vi "Setup User Messages.vi"(7 "Map Or Menu Ref":refnum<vi>, 8 "error in (no error)":errorcluster, 10 "Prev String Ref":refnum<vi>, 11 "String Ref":refnum<vi>) -> (0 "Error Out":errorcluster)   [LabVIEW 2014]
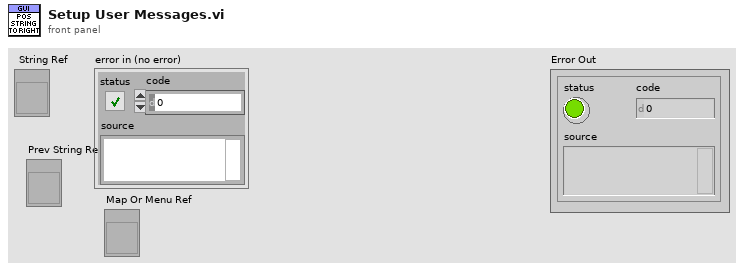
[diagram p1: front panel]
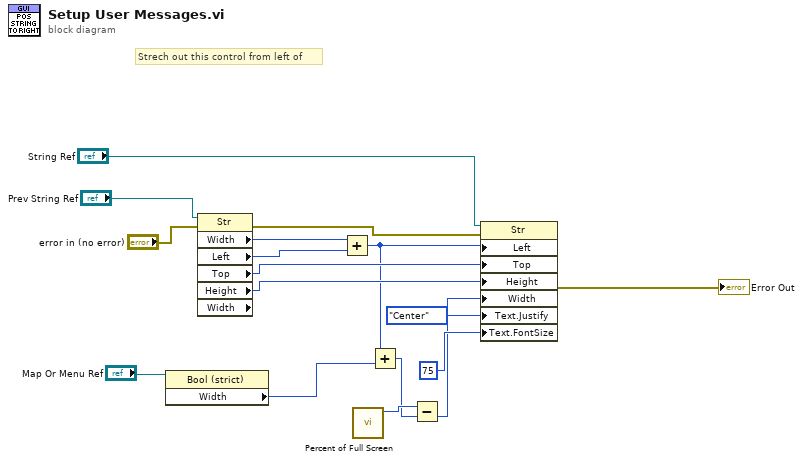
[diagram p0: block diagram]
diagram:
  # "Strech out this control from left of"
  n1 = property class="Bool (strict)"(reference="Map Or Menu Ref") -> ("Width"=w4:u32)  [unwired: 1 in, 2 out]
  n2 = property class="Str" props=["Width", "Left", "Top", "Height", "Width"](reference="Prev String Ref", error in="error in (no error)") -> (error out=w12:errorcluster, "Width"=w14:u32, "Left"=w15:i32, "Top"=w11:i32, "Height"=w10:u32)  [unwired: 2 out]
  n3 = Add(x=w14, y=w15) -> (x+y=w3:u32)
  n4 = call "Percent of Full Screen.vi"() -> ("Right"=w5:i16)  [unwired: 9 in, 2 out]
  n5 = Add(x=w3, y=w4) -> (x+y=w2:u32)
  n6 = Subtract(x=w5, y=w2) -> (x-y=w1:u32)
  n7 = property class="Str"(reference="String Ref", error in=w12, "Left"=w3, "Top"=w11, "Height"=w10, "Width"=w1, "Text.Justify"=enum16{"Left", "Center", "Right"}."Center" ("Text.Justification"), "Text.FontSize"=u32 75 ("Text.Font:Size")) -> (error out=→"Error Out":errorcluster)  [unwired: 1 out]
